vi "demo_AI ML GPU SOTA by Graiphic.vi"(11 "Stop Demo":refnum<user-event>) -> ()   [LabVIEW 2020]
panel:
  # "SOTA Suite of AI Workflows in LabVIEW! (Free for academic use)\n\nSOTA, short for State-Of-The-Art, is a suite of tools designed to simplify AI workflows by unifying key development stages. Its toolkits, particularly the Deep Learning Toolkit and the Computer Vision Toolkit, harness the power of LabVIEW to provide an intuitive graphical interface. \nhttps://graiphic.io/"
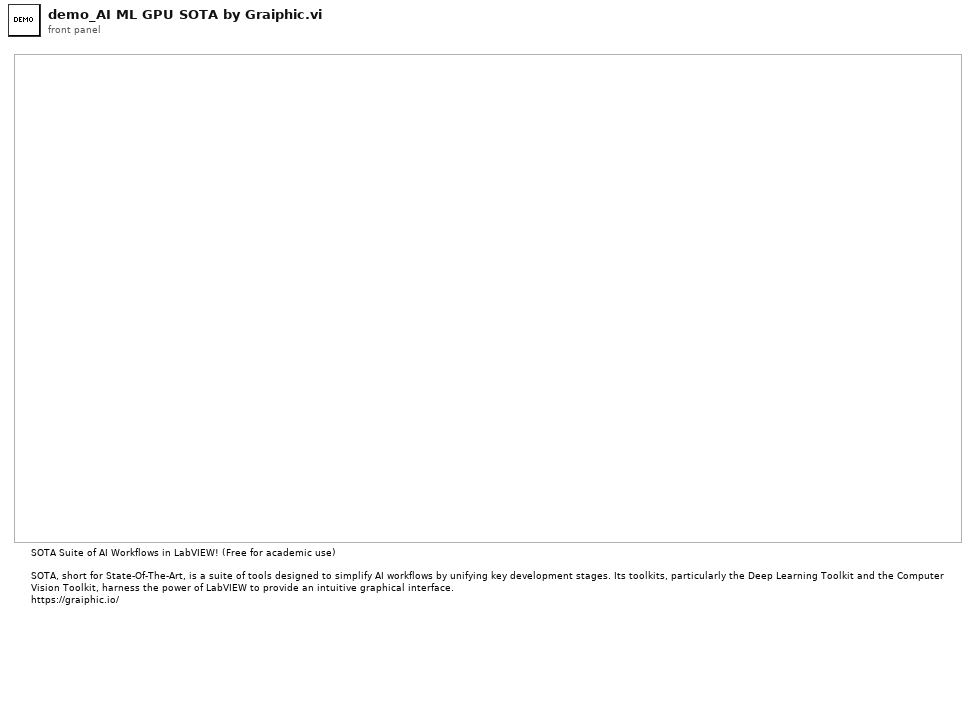
[diagram p1: front panel]
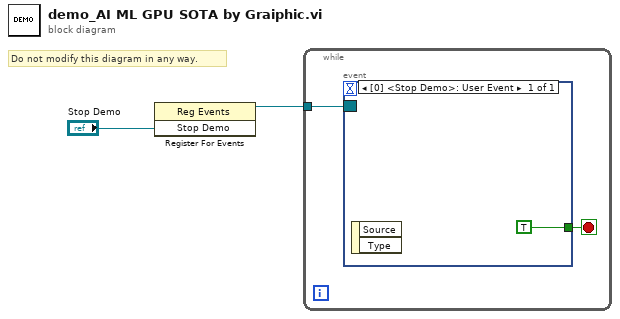
[diagram p0: block diagram]
diagram:
  # "Do not modify this diagram in any way."
  n1 = register-events("Stop Demo") -> (reference out=w1:refnum<event-registration>)  [unwired: 2 in, 1 out]
  n2 = while {
    tunnel: w1 -> [w4]
    stop <- w3 stop-if-true
    n3 = event shown="[0] <Stop Demo>: User Event" {
      selector: w4 -> [_]
      dyn-events: _ -> [_]
      timeout: _ -> [_]
      tunnel: [TRUE] -> w3
      event User Event {
        n4 = event-data() -> ()  [unwired: 1 in, 2 out]
      }
    }
  }
